vi "NoBottomLine.vi"(1 "Value in":i32[](array[numeric]), 2 "ItemNames in":string[][](array[string])) -> (0 "no bottom?":bool)   [LabVIEW 2021]
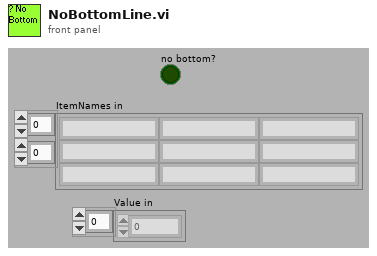
[diagram p1: front panel]
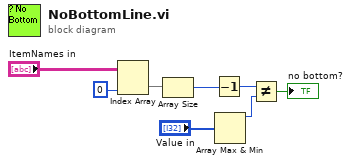
[diagram p0: block diagram]
diagram:
  n1 = Index Array(array="ItemNames in", index (col)=0 ("disabled index (col)")) -> (element=w5:string[])  [unwired: 1 in]
  n2 = Array Size(array=w5) -> (size(s)=w3:i32)
  n3 = Decrement(x=w3) -> (x-1=w7:i32)
  n4 = Array Max & Min(array="Value in") -> (max value=w8:i32)  [unwired: 3 out]
  n5 = Not Equal?(x=w7, y=w8) -> (x != y?=→"no bottom?":bool)
